vi "D-Link Colour Tracking.vi"() -> ()   [LabVIEW 2012]
uses:
  <vilib>/vision/NI_Vision_Development_Module.lvlib
  <vilib>/httpClient/LabVIEWHTTPClient.lvlib
panel:
  out "Straight Edges":T1(array[cluster]) {"Point2 (Real-World)"."Y" format="%.2f"; "Point2 (Real-World)"."X" format="%.2f"; "Point1 (Real-World)"."Y" format="%.2f"; "Point1 (Real-World)"."X" format="%.2f"; "Point2 (Pixels)"."Y" format="%.2f"; "Point2 (Pixels)"."X" format="%.2f"; "Point1 (Pixels)"."Y" format="%.2f"; "Point1 (Pixels)"."X" format="%.2f"}
  out "Number of Edges":i32
  out "Edges Coordinates":cluster{"X":sgl, "Y":sgl}[](array[cluster]) {"Y" format="%.2f"; "X" format="%.2f"}
  out "tim":u32
  out "Camera":T2(plugin-control)
  out "Particle Measurements (Pixels)":dbl[][](array[numeric]) format="%.2f"
  in  "Blue or Luma or Val or Inten Range":cluster{"Lower value":i32, "Upper value":i32}={"Lower value"=10, "Upper value"=179}
  in  "Green or Sat Range":cluster{"Lower value":i32, "Upper value":i32}={"Lower value"=20, "Upper value"=200}
  in  "Red or Hue Range":cluster{"Lower value":i32, "Upper value":i32}={"Lower value"=0, "Upper value"=200}
  in  "stop":bool
  out "BW Image":T2(plugin-control)
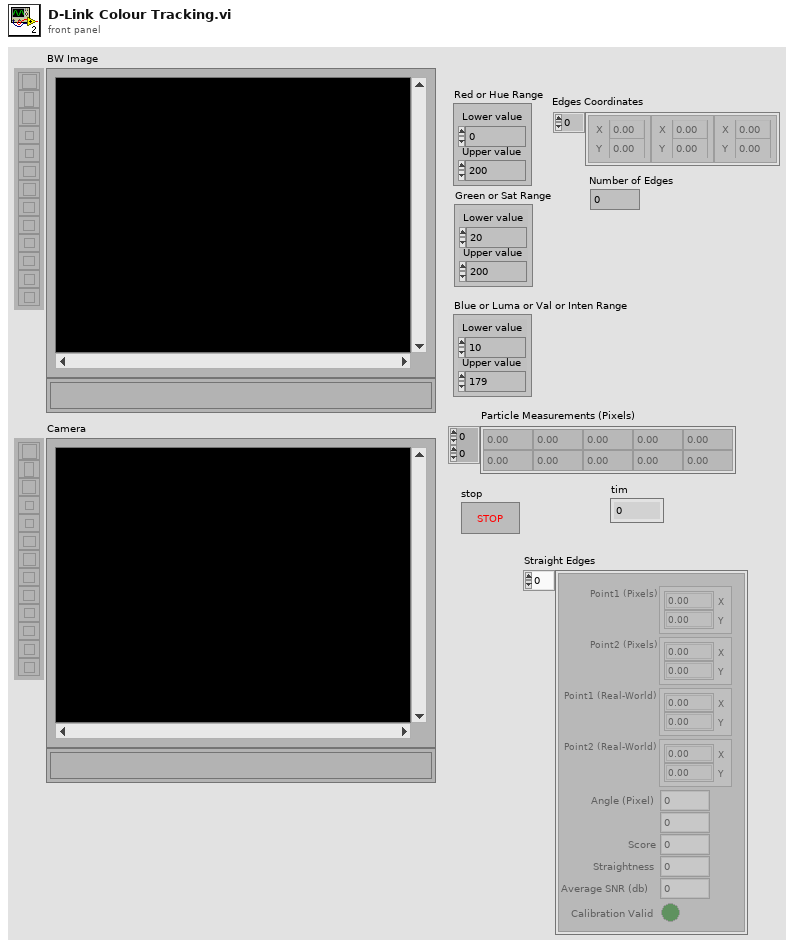
[diagram p1: front panel]
types:
  T1 = cluster{"Point1 (Pixels)":cluster{"X":sgl, "Y":sgl}, "Point2 (Pixels)":cluster{"X":sgl, "Y":sgl}, "Point1 (Real-World)":cluster{"X":sgl, "Y":sgl}, "Point2 (Real-World)":cluster{"X":sgl, "Y":sgl}, "Angle (Pixel)":dbl, "Angle (Real-World)":dbl, "Score":dbl, "Straightness":dbl, "Average SNR (db)":dbl, "Calibration Valid":bool}[]
  T2 = typedef "IMAQ Image.ctl" = refnum<image>
  T3 = cluster{"Number of Lines":i32, "Type":enum32{"First Edge Rake", "Best Edge Rake", "Hough Edge Rake", "First Edge Projection", "Best Edge Projection"}, "Min. Score":dbl, "Max. Score":dbl, "Orientation":dbl, "Angle Range":dbl, "Angle Tolerance":dbl, "Step Size":u32, "Min. SNR (db)":dbl, "Min. Points (%)":dbl, "Hough Iterations":i32}
  T4 = cluster{"Edge Polarity":u32, "Kernel Size":u32, "Width":u32, "Minimum Edge Strength":sgl, "Interpolation Type":enum32{"Zero Order", "Bilinear", "Quadratic", "Cubic", "Bilinear Fixed"}, "Data Processing Method":enum32{"Average", "Median"}}
  T5 = cluster{"Global Rectangle":i32[], "Contours":cluster{"ID":enum32{"External", "Internal"}, "Type":u32, "Coordinates":i32[]}[]}
  T6 = typedef "Image Type" = u32
  T7 = typedef "LabVIEWHTTPClient.lvlib/ClientHandle.ctl" = refnum<k1>
  T8 = enum16{"Get First Edge", "Get First + Last Edge", "Get All Edges"}
  T9 = cluster{"Level Type":enum32{"Absolute Value", "Relative value"}, "Threshold Level":i32, "Hysteresis":i32}
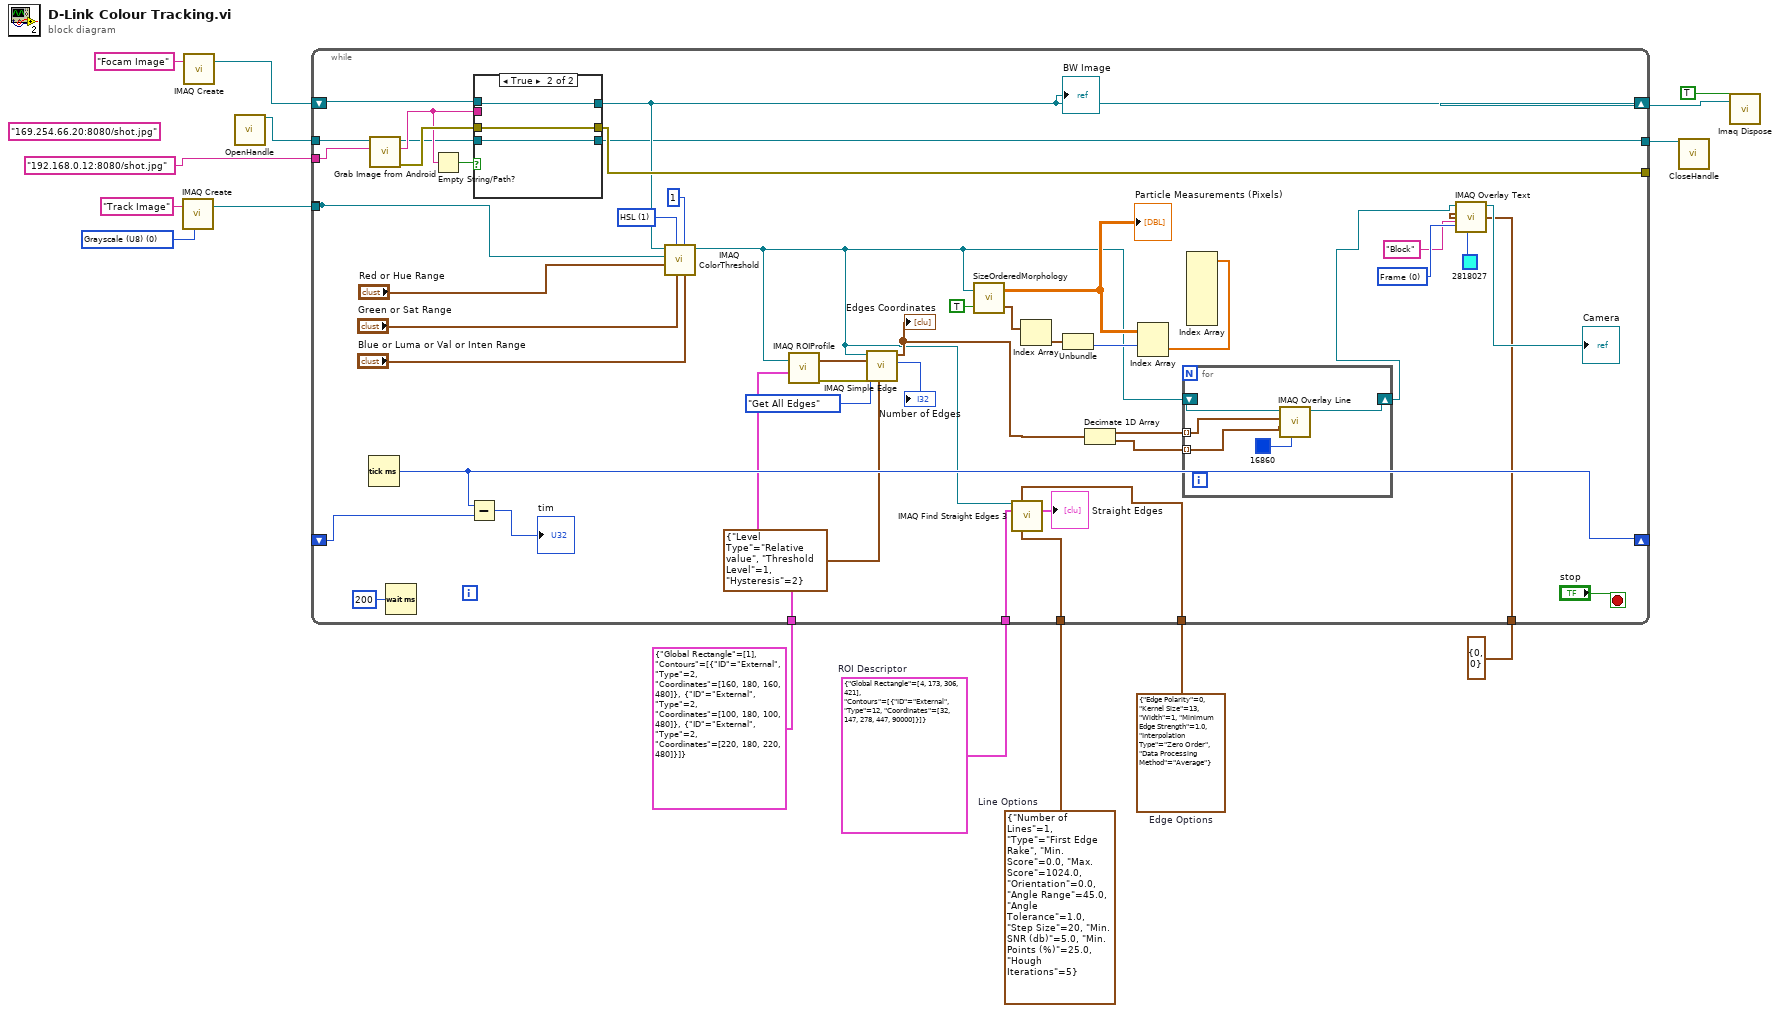
[diagram p0: block diagram]
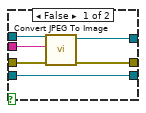
[diagram p2: hidden frame]
diagram:
  w3 = T3 {"Number of Lines"=1, "Type"=enum."First Edge Rake", "Min. Score"=0.0, "Max. Score"=1024.0, "Orientation"=0.0, "Angle Range"=45.0, "Angle Tolerance"=1.0, "Step Size"=20, "Min. SNR (db)"=5.0, "Min. Points (%)"=25.0, "Hough Iterations"=5}  # Line Options
  w2 = T4 {"Edge Polarity"=0, "Kernel Size"=13, "Width"=1, "Minimum Edge Strength"=1.0, "Interpolation Type"=enum."Zero Order", "Data Processing Method"=enum."Average"}  # Edge Options
  w1 = T5 {"Global Rectangle"=[4, 173, 306, 421], "Contours"=[{"ID"=enum."External", "Type"=12, "Coordinates"=[32, 147, 278, 447, 90000]}]}  # ROI Descriptor
  w11 = T6 0 items=["Grayscale (U8)", "Grayscale (I16)", "Grayscale (SGL)", "Complex (CSG)", "RGB (U32)", "HSL (U32)", "RGB (U64)", "Grayscale (U16)"] ("Image Type")
  (unwired) "169.254.66.20:8080/shot.jpg"
  n1 = call "IMAQ Create"("Image Name"="Track Image", "Image Type"=w11) -> ("New Image"=w12:T2)  [unwired: 3 in, 1 out]
  n2 = call "IMAQ Create"("Image Name"="Focam Image") -> ("New Image"=w13:T2)  [unwired: 4 in, 1 out]
  n3 = call <vilib>:"OpenHandle.vi"() -> ("client handle out"=w7:T7)  [unwired: 14 in, 1 out]
  n4 = while {
    tunnel: [w52] -> _
    tunnel: w12 -> [w52]
    tunnel: "192.168.0.12:8080/shot.jpg" -> [w39]
    tunnel: [w59] -> _
    shift-right: [w41] -> w10
    shift-left: w13 -> [w62]
    tunnel: cluster{"X":i32, "Y":i32} {"X"=0, "Y"=0} ("Origin") -> [w25]
    shift-right: [w42] -> _
    shift-left: _ -> [w44]
    tunnel: w7 -> [w38]
    tunnel: [w36] -> w6
    tunnel: T5 {"Global Rectangle"=[1], "Contours"=[{"ID"=enum."External", "Type"=2, "Coordinates"=[160, 180, 160, 480]}, {"ID"=enum."External", "Type"=2, "Coordinates"=[100, 180, 100, 480]}, {"ID"=enum."External", "Type"=2, "Coordinates"=[220, 180, 220, 480]}]} ("ROI Descriptor") -> [w26]
    tunnel: w3 -> [w18]
    tunnel: w2 -> [w17]
    tunnel: w1 -> [w16]
    stop <- "stop" stop-if-true
    w34 = u32 0 items=["Frame", "Fill", "Highlight"] ("Drawing Mode (Frame)")
    w55 = u16 1 items=["RGB", "HSL", "HSV", "HSI"] ("Color Mode")
    n5 = Tick Count (ms)() -> (millisecond timer value=w42:u32)
    n6 = call "Grab Image from Android.vi"("url"=w39, "client handle"=w38) -> ("error out"=w60:errorcluster, "data out"=w40:string, "client handle out"=w37:T7)  [unwired: 7 in]
    n7 = Wait (ms)(milliseconds to wait=u32 200) -> ()  [unwired: 1 out]
    n8 = Empty String/Path?(string/path=w40) -> (empty?=w61:bool)
    n9 = Subtract(x=w42, y=w44) -> (x-y=→"tim":u32)
    n10 = case shown="True" w61 {
      tunnel: w62 -> [w73 w75]
      tunnel: w60 -> [w72 w76]
      tunnel: [w71 w76] -> w59
      tunnel: [w70 w75] -> w41
      tunnel: w40 -> [w69 _]
      tunnel: w37 -> [w68 w74]
      tunnel: [w68 w74] -> w36
      frame False {
        n11 = call "Convert JPEG To Image.vi"("error in"=w72, "Compressed Image"=w69, "Image In"=w73) -> ("error out"=w71:errorcluster, "Image Out"=w70:T2)  [unwired: 7 in]
      }
      frame True {
      }
    }
    "BW Image" <- w41
    n12 = call "IMAQ ColorThreshold"("Blue or Luma or Val or Inten Range"="Blue or Luma or Val or Inten Range", "Replace Value"=1, "Green or Sat Range"="Green or Sat Range", "Color Mode"=w55, "Red or Hue Range"="Red or Hue Range", "Image Dst"=w52, "Image Src"=w41) -> ("Image Dst Out"=w20:T2)  [unwired: 3 in, 1 out]
    n13 = call "IMAQ ROIProfile"("ROI Descriptor"=w26, "Image"=w20) -> ("error out"=w27:errorcluster, "Pixel Coordinates"=w28:cluster{"X":u32, "Y":u32}[])  [unwired: 2 in, 3 out]
    n14 = call "IMAQ Simple Edge"("Threshold Parameters"=T9 {"Level Type"=enum."Relative value", "Threshold Level"=1, "Hysteresis"=2}, "error in (no error)"=w27, "Process"=T8."Get All Edges", "Pixel Coordinates"=w28, "Image Src"=w20) -> ("Number of Edges"=→"Number of Edges":i32, "Edges Coordinates"=w23:cluster{"X":sgl, "Y":sgl}[])  [unwired: 4 in, 1 out]
    "Edges Coordinates" <- w23
    n15 = call "SizeOrderedMorphology.vi"("Green"=TRUE, "Image Dst Out"=w20) -> ("Sort Array"=w49:cluster{"Numeric":dbl, i32}[], "Particle Measurements (Pixels)"=w45:dbl[][])
    "Particle Measurements (Pixels)" <- w45
    n16 = call "IMAQ Find Straight Edges 3"("Image"=w20, "Edge Options"=w17, "ROI Descriptor"=w16, "Line Options"=w18) -> ("Straight Edges"=→"Straight Edges":T1)  [unwired: 7 in, 4 out]
    n17 = Index Array(array=w49) -> (element=w48:cluster{"Numeric":dbl, i32})  [unwired: 1 in]
    n18 = Unbundle(w48) -> (w47:i32)  [unwired: 1 out]
    n19 = Decimate 1D Array(w23) -> (w22:cluster{"X":sgl, "Y":sgl}[], w21:cluster{"X":sgl, "Y":sgl}[])
    n20 = Index Array(array=w45, index (row)=w47) -> (element=w46:dbl[])  [unwired: 1 in]
    n21 = for {
      shift-right: [w66] -> w24
      shift-left: w20 -> [w67]
      tunnel: w22 -> [w65] mode=indexing
      tunnel: w21 -> [w64] mode=indexing
      n22 = call "IMAQ Overlay Line"("Color"=u32 16860, "End Point"=w64, "Start Point"=w65, "Image"=w67) -> ("Image Out"=w66:T2)  [unwired: 6 in, 1 out]
    }
    n23 = Index Array(array=w46) -> ()  [unwired: 7 in, 7 out]
    n24 = call "IMAQ Overlay Text"("BG Color (Transparent)"=w34, "Text Color (black)"=u32 2818027 ("Color"), "String"="Block", "Origin"=w25, "Image"=w24) -> ("Image Out"=→"Camera":T2)  [unwired: 5 in, 1 out]
  }
  n25 = call <vilib>:"CloseHandle.vi"("client handle"=w6) -> ()  [unwired: 14 in, 1 out]
  n26 = call "Imaq Dispose"("All Images? (No)"=TRUE, "Image"=w10) -> ()  [unwired: 4 in, 1 out]
